vi "RSZVB Trace Export Data Ports.vi"(0 "VISA session":refnum<visa-resource-name>, 1 "Port 1 (1)":i32=1, 2 "Port 3 (3)":i32=3, 5 "Channel (1)":i32=1, 7 "File Name (\"Trc1.s1p\")":string="Trc1.s1p", 9 "Export Data (Complex Values)":i32(ring) items=["Complex Values", "Linear magnitude and phase", "dB-magnitude and phase"], 11 "error in (no error)":errorcluster {"code" format="%.0x"}, 12 "Port 2 (2)":i32=2, 13 "Port 4 (4)":i32=4) -> (4 "dup VISA session":refnum<visa-resource-name>, 15 "error out":errorcluster {"code" format="%.0x"})   [LabVIEW 2011]
doc: "This VI stores the trace data to a Touchstone file for the specified ports. The Touchstone file (.s<n>p where <n> is the number of ports) contains a full set of <n>2 single-ended S-parameters for the selected ports.\n\nNote(s):\n\n(1) Traces are created using the CALCulte<Ch>:PARameter:SDEFine... command.\n\n(2) The VI fails unless the following conditions are met: \n\n- For a one-port Touchstone file, the reflection coefficient for the specified port (e.g. S11 for port no. 1) must be measured. If a full one-port system error correction is available for the specified port, it is also possible to export transmission parameters that are related to the calibrated port (e.g. S12 or S21 for port no. 1).\n\n- For a multiport Touchstone file, a full multiport system error correction must be available. It is not necessary to measure the full set of S-parameters. Moreover, if the port configuration contains balanced ports, the Touchstone file will contain the converted single-ended S-parameters.\n\nRemote-control command(s):\nMMEMory:STORe:TRACe:PORTs"
uses:
  _utility/RSZVB Global Data.vi
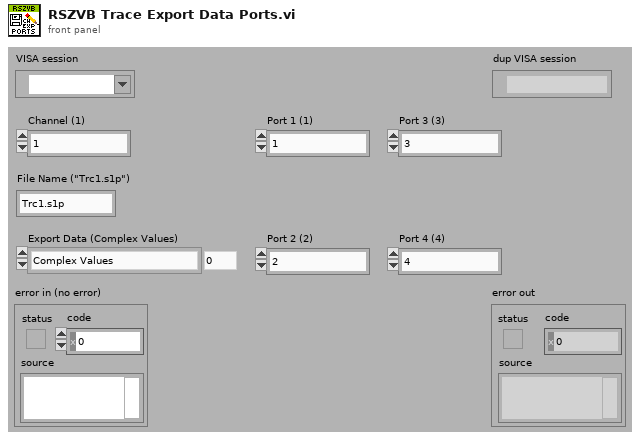
[diagram p1: front panel]
types:
  T1 = cluster{"Error Checking (T: On)":bool, "Installed Options":string[], "Data Valid?":bool, "Ports":i32, "Model":string[], "Option Checking (T: On)":bool}[]
  T2 = cluster{"Error Checking (T: On)":bool, "Installed Options":string[], "Data Valid?":bool, "Ports":i32, "Model":string[], "Option Checking (T: On)":bool}
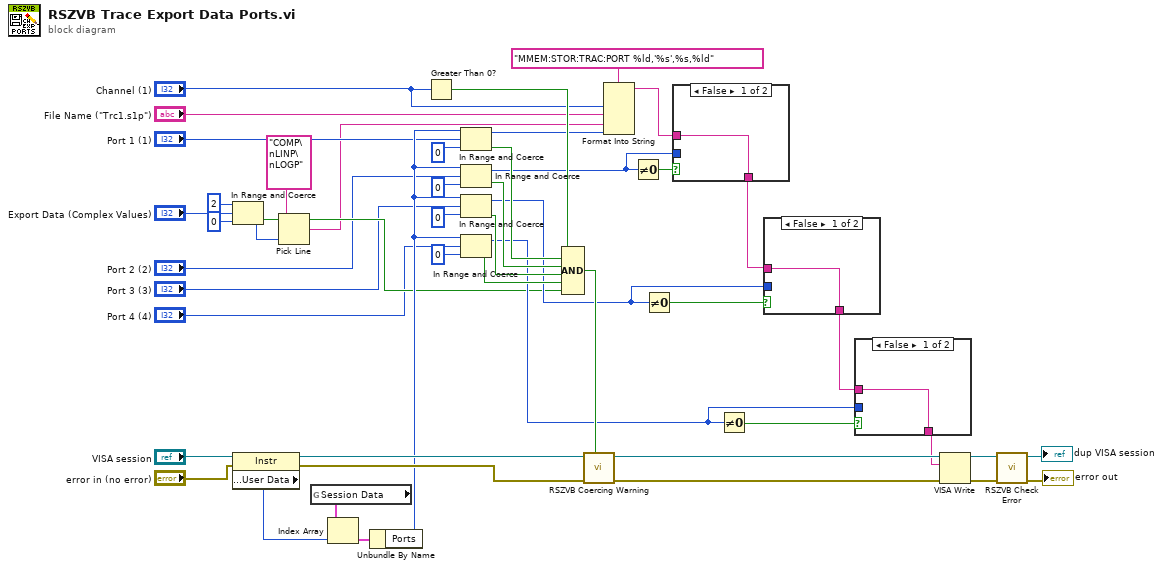
[diagram p0: block diagram]
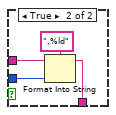
[diagram p2: hidden frame]
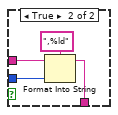
[diagram p3: hidden frame]
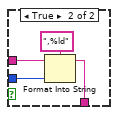
[diagram p4: hidden frame]
diagram:
  n1 = In Range and Coerce(upper limit=2 ("lower limit"), x="Export Data (Complex Values)", lower limit=0) -> (coerced(x)=w7:i32, In Range?=w6:bool)
  n2 = property class="Instr"(reference="VISA session", error in="error in (no error)") -> (reference out=w41:refnum<visa-resource-name>, error out=w42:errorcluster, "General Settings:User Data"=w21:u32)
  n3 = Pick Line(multi-line string="COMP\nLINP\nLOGP", line index=w7) -> (output string=w2:string)  [unwired: 1 in]
  n4 = global read "RSZVB Global Data.vi" "Session Data"() -> (w43:T1)
  n5 = Index Array(array=w43, index=w21) -> (element=w44:T2)
  n6 = Unbundle By Name(w44) -> ("Ports"=w30:i32)
  n7 = Greater Than 0?(x="Channel (1)") -> (x > 0?=w45:bool)
  n8 = In Range and Coerce(upper limit=w30, x="Port 1 (1)", lower limit=0) -> (coerced(x)=w9:i32, In Range?=w37:bool)
  n9 = In Range and Coerce(upper limit=w30, x="Port 2 (2)", lower limit=0) -> (coerced(x)=w24:i32, In Range?=w36:bool)
  n10 = In Range and Coerce(upper limit=w30, x="Port 3 (3)", lower limit=0) -> (coerced(x)=w22:i32, In Range?=w35:bool)
  n11 = In Range and Coerce(upper limit=w30, x="Port 4 (4)", lower limit=0) -> (coerced(x)=w23:i32, In Range?=w34:bool)
  n12 = Compound Arithmetic op=AND(w45, w37, w36, w35, w34, w6) -> (w46:bool)
  n13 = call "RSZVB Coercing Warning.vi"("In Range?"=w46, "error in (no error)"=w42, "VISA session"=w41) -> ("error out"=w47:errorcluster, "dup VISA session"=w48:refnum<visa-resource-name>)  [unwired: 7 in]
  n14 = Format Into String(format string="MMEM:STOR:TRAC:PORT %ld,'%s',%s,%ld", "Channel (1)", "File Name (\"Trc1.s1p\")", w2, w9) -> (resulting string=w31:string)  [unwired: 2 in, 1 out]
  n15 = Not Equal To 0?(x=w24) -> (x != 0?=w32:bool)
  n16 = Not Equal To 0?(x=w22) -> (x != 0?=w29:bool)
  n17 = case shown="False" w32 {
    tunnel: w31 -> [w50 w54]
    tunnel: w24 -> [_ w52]
    tunnel: [w50 w51] -> w27
    frame False {
    }
    frame True {
      n18 = Format Into String(format string=",%ld", initial string=w54, w52) -> (resulting string=w51:string)  [unwired: 1 in, 1 out]
    }
  }
  n19 = Not Equal To 0?(x=w23) -> (x != 0?=w28:bool)
  n20 = case shown="False" w29 {
    tunnel: w27 -> [w55 w59]
    tunnel: w22 -> [_ w57]
    tunnel: [w55 w56] -> w26
    frame False {
    }
    frame True {
      n21 = Format Into String(format string=",%ld", initial string=w59, w57) -> (resulting string=w56:string)  [unwired: 1 in, 1 out]
    }
  }
  n22 = case shown="False" w28 {
    tunnel: w26 -> [w60 w64]
    tunnel: w23 -> [_ w62]
    tunnel: [w60 w61] -> w25
    frame False {
    }
    frame True {
      n23 = Format Into String(format string=",%ld", initial string=w64, w62) -> (resulting string=w61:string)  [unwired: 1 in, 1 out]
    }
  }
  n24 = VISA Write(VISA resource name=w48, write buffer=w25, error in (no error)=w47) -> (VISA resource name out=w16:refnum<visa-resource-name>, error out=w15:errorcluster)  [unwired: 1 out]
  n25 = call "RSZVB Check Error.vi"("error in (no error)"=w15, "VISA session"=w16) -> ("error out"=→"error out":errorcluster, "dup VISA session"=→"dup VISA session":refnum<visa-resource-name>)  [unwired: 8 in]
